vi "CarNOCheck.vi"(10 "CARNO":i32) -> (2 "CarNO":string)   [LabVIEW 2014]
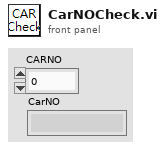
[diagram p1: front panel]
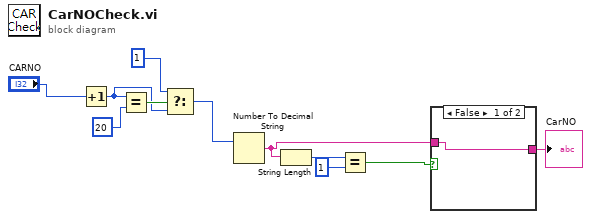
[diagram p0: block diagram]
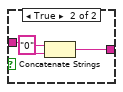
[diagram p2: hidden frame]
diagram:
  n1 = Increment(x="CARNO") -> (x+1=w8:i32)
  n2 = Equal?(x=w8, y=20) -> (x = y?=w10:bool)
  n3 = Select(t=1, s=w10, f=w8) -> (s? t:f=w7:i32)
  n4 = Number To Decimal String(number=w7) -> (decimal integer string=w2:string)  [unwired: 1 in]
  n5 = String Length(string=w2) -> (length=w5:i32)
  n6 = Equal?(x=w5, y=1) -> (x = y?=w3:bool)
  n7 = case shown="False" w3 {
    tunnel: w2 -> [w12 w15]
    tunnel: [w12 w13] -> w1
    frame False {
    }
    frame True {
      n8 = Concatenate Strings("0" ("string"), w15) -> (w13:string)
    }
  }
  "CarNO" <- w1
